vi "Close_Game.vi"(0 "VI_In":refnum<vi>, 11 "Error_In":errorcluster) -> (15 "Error_Out":errorcluster)   [LabVIEW 2023]
doc: "This VI Closes the front panel and the reference of the VI."
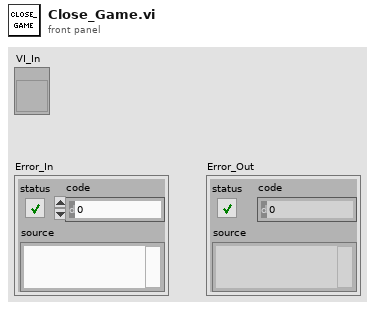
[diagram p1: front panel]
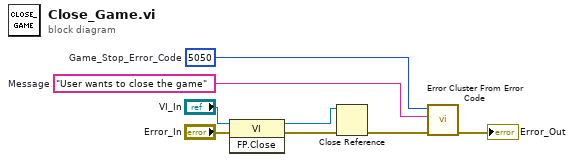
[diagram p0: block diagram]
diagram:
  w8 = "User wants to close the game"  # Message
  w7 = 5050  # Game_Stop_Error_Code
  n1 = invoke class="VI" method="FP.Close"(reference="VI_In", error in="Error_In") -> (reference out=w1:refnum<vi>, error out=w2:errorcluster)  [unwired: 1 in, 1 out]
  n2 = Close Reference(reference=w1, error in (no error)=w2) -> (error out=w5:errorcluster)
  n3 = call <vilib>:"Error Cluster From Error Code.vi"("error in (no error)"=w5, "error message (\"\")"=w8, "error code (0)"=w7) -> ("error out"=→"Error_Out":errorcluster)  [unwired: 6 in]
